vi "Unibot - State Machine Controller.vi"(3 "dt (s)":dbl=-1.0 format="%.3f", 4 "Limit":dbl=10.0, 5 "Up Optimal Gain":dbl[](array[numeric])=[-16.4615, -16.2422, -3.1287, -2.0658], 6 "Mode":T1(ring), 7 "Setpoint":dbl(knob) scale=-1.0..1.0, 8 "Enable":bool, 9 "Kill":bool, 10 "PID gains":T2={"proportional gain (Kc)"=1.0, "integral time (Ti, min)"=0.01, "derivative time (Td, min)"=0.0} {"derivative time (Td, min)" format="%.3f"; "integral time (Ti, min)" format="%.3f"; "proportional gain (Kc)" format="%.3f"}, 11 "States":dbl[](array[numeric])=[-0.0012566370614359172, -0.8117875416876026, 0.0, 0.0]) -> (0 "Status":string="Kill", 2 "Control Effort":i32(knob) scale=-1000.0..1000.0)   [LabVIEW 2012]
uses:
  Unibot - States.ctl
  <vilib>/addons/Control Design/_Implementation/CD State Feedback Controller (Single Output).vi
  <vilib>/addons/control/pid/pid.llb/PID (DBL).vi
  <vilib>/addons/Control Design/_Implementation/NI_CD_Implementation.lvlib
  <vilib>/addons/control/pid/NI_PID_pid.lvlib
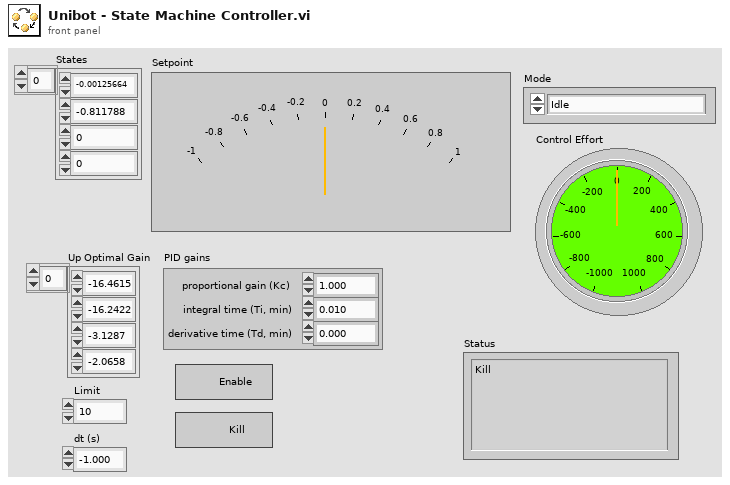
[diagram p1: front panel]
types:
  T1 = enum16{"Idle", "Linear Balance", "Proportional Balance", "PID Balance", "Emergency"}
  T2 = cluster{"proportional gain (Kc)":dbl, "integral time (Ti, min)":dbl, "derivative time (Td, min)":dbl}
  T3 = typedef "Unibot - States.ctl" = enum16{"Idle", "Balance", "Emergency"}
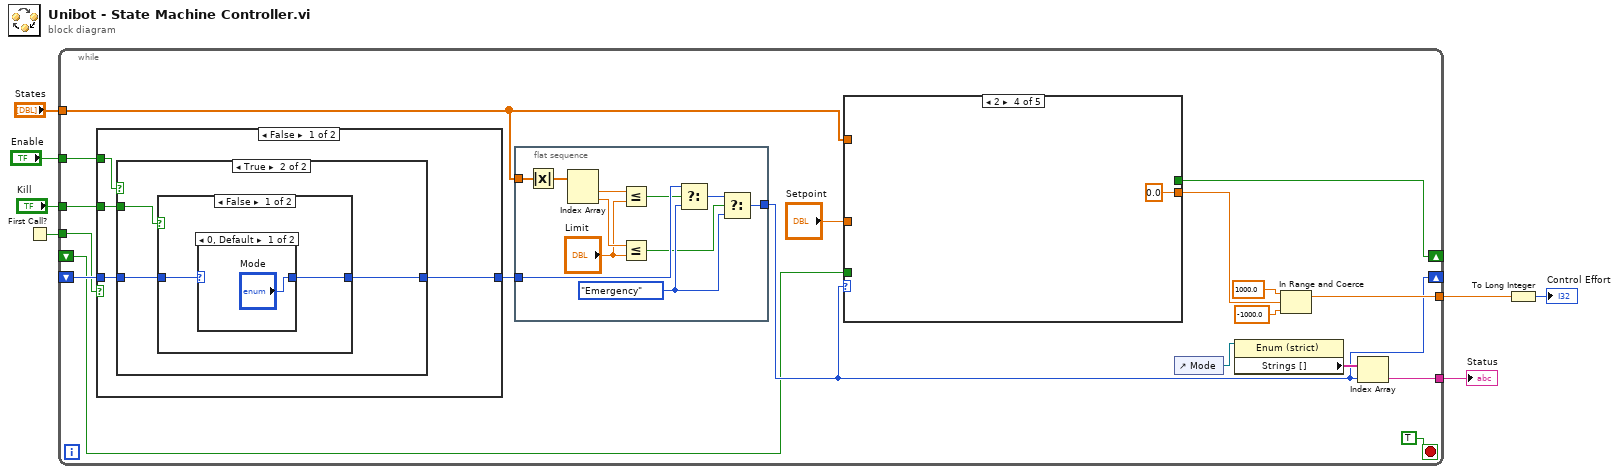
[diagram p0: block diagram]
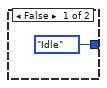
[diagram p2: hidden frame]
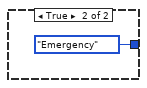
[diagram p4: hidden frame]
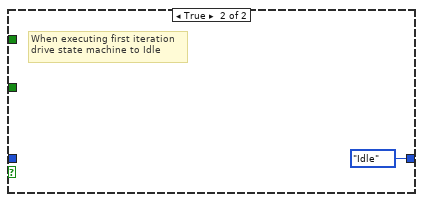
[diagram p5: hidden frame]
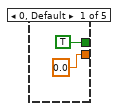
[diagram p6: hidden frame]
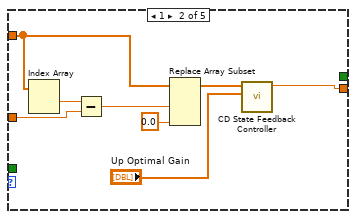
[diagram p7: hidden frame]
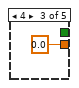
[diagram p8: hidden frame]
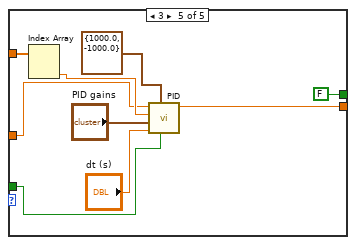
[diagram p9: hidden frame]
diagram:
  n1 = First Call?() -> (First Call?: T/F=w4:bool)
  n2 = while {
    tunnel: "States" -> [w20]
    tunnel: [w17] -> w1
    shift-right: [w13] -> _
    shift-left: _ -> [w23]
    tunnel: [w12] -> w6
    tunnel: "Kill" -> [w24]
    tunnel: w4 -> [w22]
    tunnel: "Enable" -> [w21]
    shift-right: [w10] -> _
    shift-left: _ -> [w11]
    stop <- TRUE stop-if-true
    n3 = case shown="False" w22 {
      tunnel: w24 -> [w40 _]
      tunnel: w23 -> [w39 _]
      tunnel: w21 -> [w38 _]
      tunnel: [w37 Unibot_-_States."Idle" ("Enum")] -> w19
      frame False {
        n4 = case shown="True" w38 {
          tunnel: w40 -> [_ w44]
          tunnel: w39 -> [_ w42]
          tunnel: [Unibot_-_States."Idle" ("Enum") w43] -> w37
          frame False {
          }
          frame True {
            n5 = case shown="False" w44 {
              tunnel: [w45 Unibot_-_States."Emergency" ("Enum")] -> w43
              tunnel: w42 -> [w46 _]
              frame False {
                n6 = case shown="0, Default" w46 {
                  selector: w46 -> [_ w48]
                  tunnel: ["Mode" w48] -> w45
                  frame 0, Default {
                  }
                  frame 4 {
                  }
                }
              }
              frame True {
              }
            }
          }
        }
      }
      frame True {
        # "When executing first iteration\ndrive state machine to Idle"
      }
    }
    n7 = flat-sequence {
      tunnel: w20 -> [w31]
      tunnel: w19 -> [w36]
      tunnel: [w33] -> w13
      frame #0 {
        w34 = Unibot_-_States."Emergency" ("Enum")
        n8 = Absolute Value(x=w31) -> (abs(x)=w32:dbl[])
        n9 = Index Array(array=w32) -> (element #1=w29:dbl, element #2=w30:dbl)  [unwired: 2 in]
        n10 = Less Or Equal?(x=w29, y="Limit") -> (x <= y?=w28:bool)
        n11 = Less Or Equal?(x=w30, y="Limit") -> (x <= y?=w27:bool)
        n12 = Select(t=w36, s=w28, f=w34) -> (s? t:f=w35:u16)
        n13 = Select(t=w35, s=w27, f=w34) -> (s? t:f=w33:u16)
      }
    }
    n14 = case shown="2" w13 {
      tunnel: w20 -> [_ w57 _ _ w68]
      tunnel: [0.0 w55 0.0 0.0 ("output") w69] -> w18
      tunnel: "Setpoint" -> [_ w54 _ _ w66]
      tunnel: w11 -> [_ _ _ _ w64]
      tunnel: [TRUE ("Enable") _ _ _ FALSE ("Enable")] -> w10
      frame 0, Default {
      }
      frame 1 {
        n15 = Index Array(array=w57) -> (element #1=w56:dbl)  [unwired: 2 in, 1 out]
        n16 = Subtract(x=w56, y=w54) -> (x-y=w59:dbl)
        n17 = Replace Array Subset(array=w57, new element #1=w59, new element #2=0.0 ("x")) -> (w60:dbl[])  [unwired: 2 in]
        n18 = call-poly <vilib>:"CD State Feedback Controller.vi"("Controller Gain"="Up Optimal Gain", "States"=w60) -> ("Controller Action"=w55:dbl)  [unwired: 1 in, 8 out]
      }
      frame 4 {
      }
      frame 2 {
      }
      frame 3 {
        n19 = Index Array(array=w68) -> (element #2=w67:dbl)  [unwired: 2 in, 1 out]
        n20 = call-poly <vilib>:"PID.vi"("reinitialize? (F)"=w64, "output range"=cluster{"output high":dbl, "output low":dbl} {"output high"=1000.0, "output low"=-1000.0}, "dt (s)"="dt (s)", "PID gains"="PID gains", "process variable"=w67, "setpoint"=w66) -> ("output"=w69:dbl)  [unwired: 4 in, 1 out]
      }
    }
    n21 = control-ref of="Mode"() -> (w8:refnum<vi>)
    n22 = property class="Enum (strict)"(reference=w8) -> ("Strings []"=w14:string[])  [unwired: 1 in, 2 out]
    n23 = In Range and Coerce(upper limit=1000.0, x=w18, lower limit=-1000.0) -> (coerced(x)=w17:dbl)  [unwired: 1 out]
    n24 = Index Array(array=w14, index=w13) -> (element=w12:string)
  }
  "Status" <- w6
  n25 = To Long Integer(number=w1) -> (32bit integer=→"Control Effort":i32)
